vi "EEI Lab Exps Demo.vi"() -> ()   [LabVIEW 2020]
panel:
  out "EVEN no.s while loop":i32[](array[numeric])
  out "EVEN no.s for loop":i32[](array[numeric])
  in  "even no.s":i32
  out "current time":timestamp
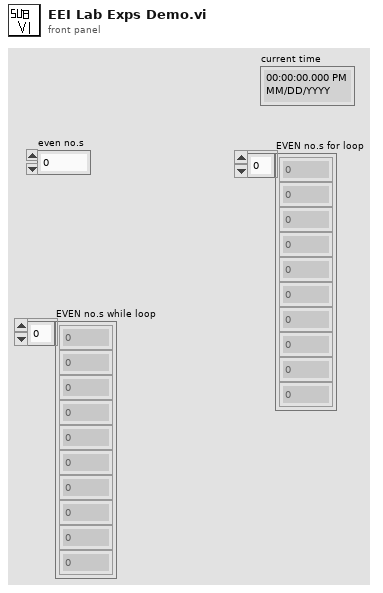
[diagram p1: front panel]
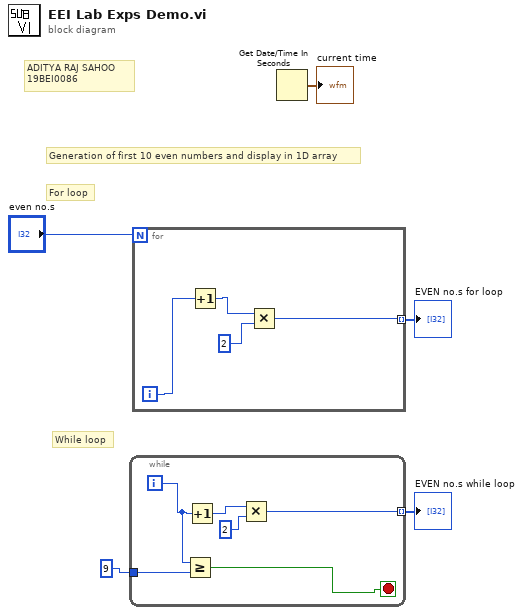
[diagram p0: block diagram]
diagram:
  # "While loop"
  # "For loop"
  # "Generation of first 10 even numbers and display in 1D array"
  # "ADITYA RAJ SAHOO\n19BEI0086"
  n1 = while {
    tunnel: 9 ("y") -> [w7]
    tunnel: [w6] -> w1 mode=indexing
    i -> [w8]
    stop <- w11 stop-if-true
    n2 = Greater Or Equal?(x=w8, y=w7) -> (x >= y?=w11:bool)
    n3 = Increment(x=w8) -> (x+1=w10:i32)
    n4 = Multiply(x=w10, y=2) -> (x*y=w6:i32)
  }
  "EVEN no.s while loop" <- w1
  n5 = for {
    N: "even no.s" -> [_]
    tunnel: [w12] -> w3 mode=indexing
    i -> [w15]
    n6 = Increment(x=w15) -> (x+1=w14:i32)
    n7 = Multiply(x=w14, y=2) -> (x*y=w12:i32)
  }
  "EVEN no.s for loop" <- w3
  n8 = Get Date/Time In Seconds() -> (seconds since 1Jan1904=→"current time":timestamp)
